vi "Acquire Image.vi"(8 "Error In":errorcluster, 11 "Acquire Data":cluster{"Image Para":T1[], "Image Path":path} {"Image Para"."set shutter(s)" min=0.001 max=3.0 step=0.001; "Image Para"."Power(Amp)" min=15 max=100}) -> (0 "Error Out":errorcluster)   [LabVIEW 2019, in "Image.lvlib"]
uses:
  Image.lvlib
  LED/SubVI/Image Para.ctl
  MiControl-E/LV Source/ImageSystem/Cradle Zyla_1117/Ctl/seletion.ctl
  Queues/Queues.lvlib
  LED/LED.lvlib
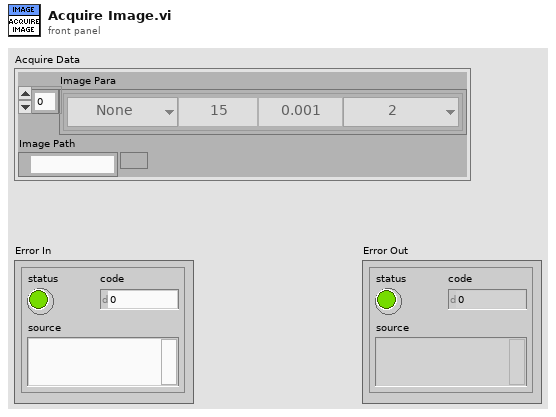
[diagram p1: front panel]
types:
  T1 = typedef "LED.lvlib/Image Para.ctl" = cluster{"Marker":T2, "Power(Amp)":u8, "set shutter(s)":dbl, "Cube":enum16{"1", "2", "3", "4", "5", "6", "7", "8"}}
  T2 = typedef "seletion.ctl" = enum16{"None", "Red", "Green", "Blue", "UV", "Green Laser", "Blue-Red", "UV-Red", "BF", "UV-IR"}
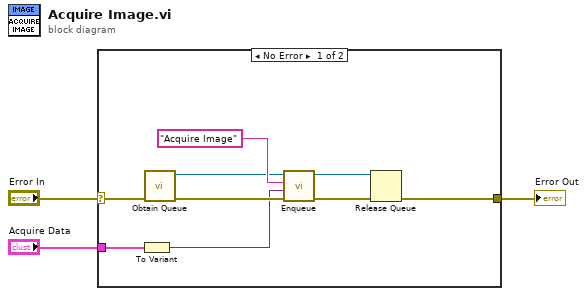
[diagram p0: block diagram]
diagram:
  n1 = case shown="No Error" "Error In" {
    selector: "Error In" -> [w8 w13]
    tunnel: [w9 w13] -> w3
    tunnel: "Acquire Data" -> [w5 _]
    frame No Error {
      n2 = To Variant(anything=w5) -> (Variant=w4:variant)
      n3 = call "Obtain Queue.vi"("Error In"=w8) -> ("Error Out"=w7:errorcluster, "Queue out"=w6:refnum<queue>)  [unwired: 9 in]
      n4 = call "Enqueue.vi"("Error In"=w7, "Data"=w4, "State"="Acquire Image", "Queue in"=w6) -> ("Error Out"=w11:errorcluster, "Queue out"=w10:refnum<queue>)  [unwired: 6 in]
      n5 = Release Queue(queue=w10, error in (no error)=w11) -> (error out=w9:errorcluster)  [unwired: 1 in, 2 out]
    }
    frame Error {
    }
  }
  "Error Out" <- w3
